vi "Array - Write Age.vi"(8 "error in (no error)":errorcluster, 10 "Ages":dbl[](array[numeric]), 11 "Input Array":refnum<class "myClass.lvclass">[](array[class])=[refnum, refnum]) -> (0 "error out":errorcluster, 3 "Output Array":refnum<class "myClass.lvclass">[](array[class]))   [LabVIEW 2013]
uses:
  ClassDefinitions/SimpleClassWithProperties/myClass.lvclass
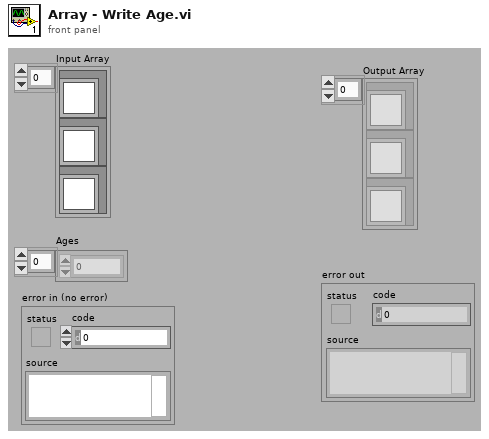
[diagram p1: front panel]
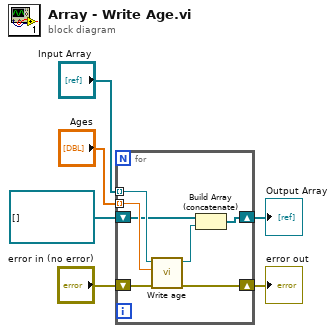
[diagram p0: block diagram]
diagram:
  n1 = for {
    tunnel: "Input Array" -> [w13] mode=indexing
    tunnel: "Ages" -> [w12] mode=indexing
    shift-right: [w9] -> w4
    shift-left: refnum<class "myClass.lvclass">[] [] ("Input Array") -> [w11]
    shift-right: [w8] -> w2
    shift-left: "error in (no error)" -> [w7]
    n2 = call-dynamic "Write age.vi"("error in (no error)"=w7, "age"=w12, "myClass in"=w13) -> ("error out"=w8:errorcluster, "myClass out"=w10:refnum<class "myClass.lvclass">)  [unwired: 7 in]
    n3 = Build Array (concatenate)(w11, w10) -> (w9:refnum<class "myClass.lvclass">[])
  }
  "Output Array" <- w4
  "error out" <- w2
